vi "Explain Error.vi"(6 "Explanation":string, 9 "error in (no error)":errorcluster, 10 "Detected? (F)":bool) -> (1 "error out":errorcluster)   [LabVIEW 2011]
doc: "Adds explanatory information to an error if detected.\n\n\nVersion 1.0 - 02/13/2013\n\nPhaeron, Inc.\nwww.phaeron.com\ninfo@phaeron.com"
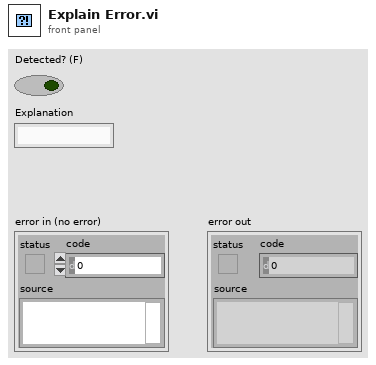
[diagram p1: front panel]
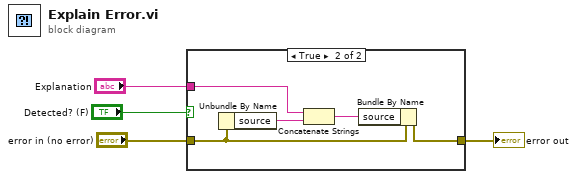
[diagram p0: block diagram]
diagram:
  n1 = case shown="True" "Detected? (F)" {
    tunnel: [w5 w10] -> w4
    tunnel: "error in (no error)" -> [w5 w9]
    tunnel: "Explanation" -> [_ w6]
    frame False {
    }
    frame True {
      n2 = Unbundle By Name(w9) -> ("source"=w8:string)
      n3 = Concatenate Strings(w6, w8) -> (w7:string)
      n4 = Bundle By Name(cluster=w9, "source"=w7) -> (w10:errorcluster)
    }
  }
  "error out" <- w4
